vi "TempratureSensing.vi"() -> ()   [LabVIEW 2019]
panel:
  out "Temp":dbl
  out "Temprature  Meter":dbl(knob) scale=0.0..400.0
  out "LOW":bool
  out "Modreate":bool
  out "High":bool
  in  "Temprature":dbl(slide) scale=0.0..400.0
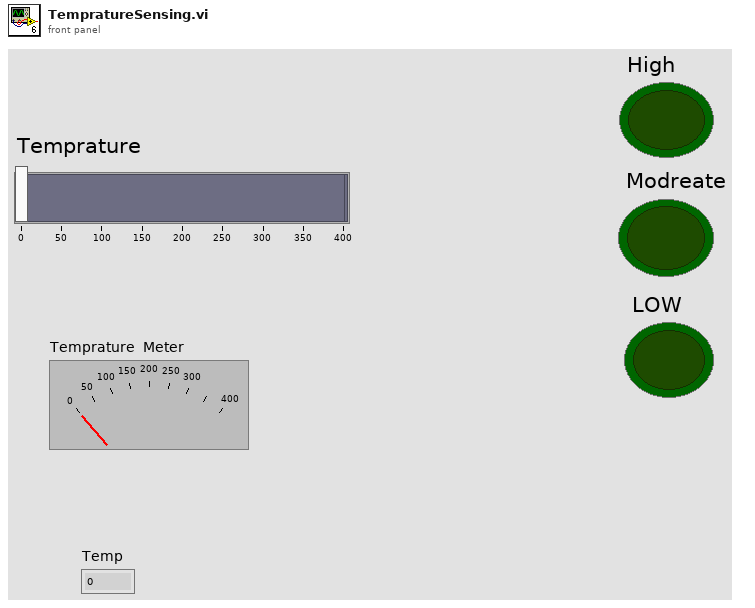
[diagram p1: front panel]
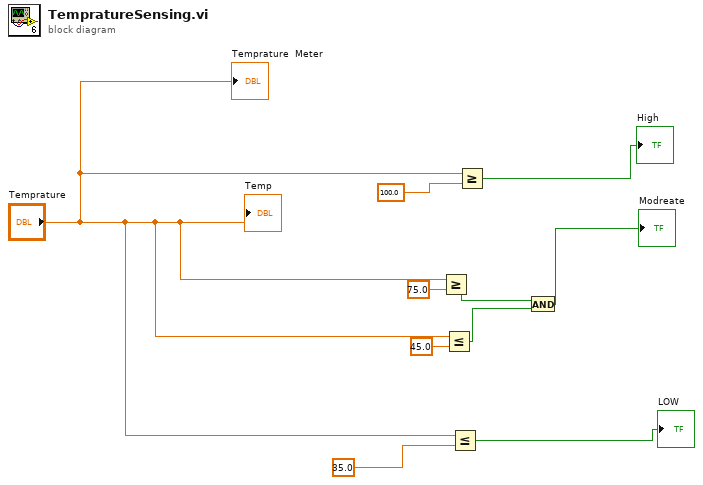
[diagram p0: block diagram]
diagram:
  n1 = Greater Or Equal?(x="Temprature", y=75.0) -> (x >= y?=w8:bool)
  n2 = Less Or Equal?(x="Temprature", y=45.0) -> (x <= y?=w7:bool)
  n3 = Less Or Equal?(x="Temprature", y=35.0) -> (x <= y?=→"LOW":bool)
  n4 = Greater Or Equal?(x="Temprature", y=100.0) -> (x >= y?=→"High":bool)
  n5 = And(x=w8, y=w7) -> (x .and. y?=→"Modreate":bool)
  "Temprature  Meter" <- "Temprature"
  "Temp" <- "Temprature"
